vi "UI extra controls.vi"() -> ()   [LabVIEW 2022 SP3]
panel:
  in  "Launch Recipe Editor":bool
  in  "Launch DAQ Config":bool
  in  "Combined View":bool
  in  "Config. Head Compensation":bool
  in  "Match Compensation Settings":bool
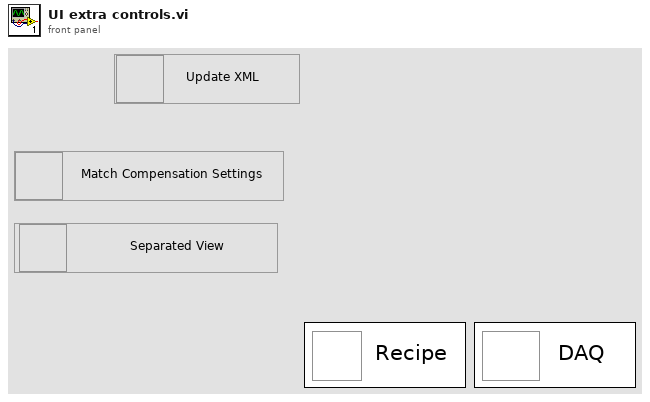
[diagram p1: front panel]
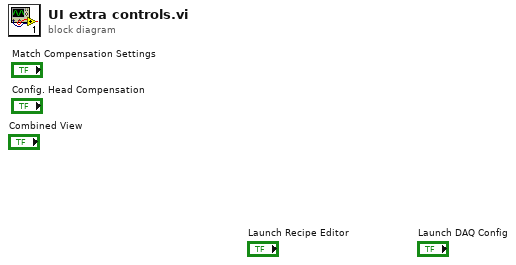
[diagram p0: block diagram]
diagram:
